vi "check_min_max_rules.vi"(10 "rules list":string[][](array[string])) -> (0 "empty/wrong?":bool=TRUE, 1 "message":string, 2 "min_length":string, 3 "max_length":string)   [LabVIEW 2024]
panel:
  # "max"
  # "min"
  # "lit when empty/wrong"
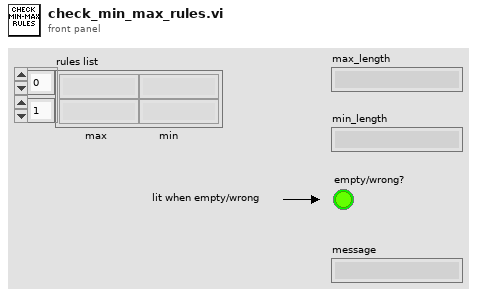
[diagram p1: front panel]
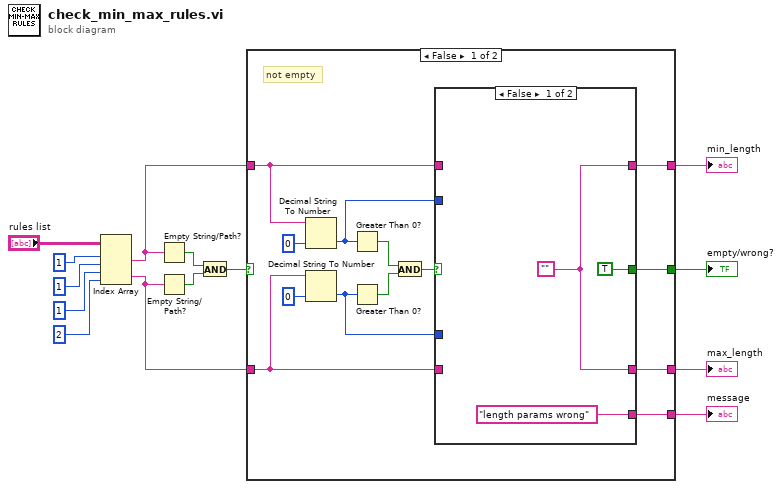
[diagram p0: block diagram]
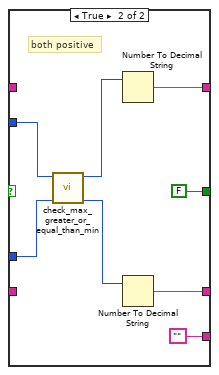
[diagram p2: hidden frame]
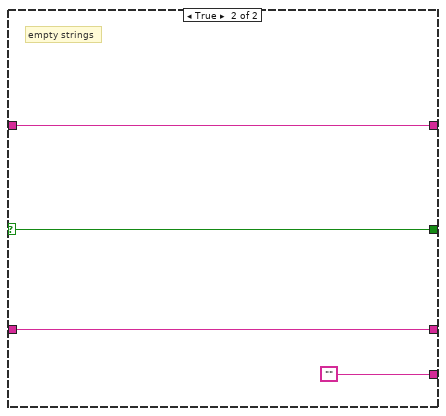
[diagram p3: hidden frame]
diagram:
  n1 = Index Array(array="rules list", index (row) #1=1 ("index"), index (col) #1=1 ("index"), index (row) #2=1 ("index"), index (col) #2=2 ("index")) -> (element #1=w9:string, element #2=w8:string)
  n2 = Empty String/Path?(string/path=w9) -> (empty?=w12:bool)
  n3 = Empty String/Path?(string/path=w8) -> (empty?=w11:bool)
  n4 = And(x=w12, y=w11) -> (x .and. y?=w10:bool)
  n5 = case shown="False" w10 {
    selector: w10 -> [_ w41]
    tunnel: w9 -> [w19 w40]
    tunnel: w8 -> [w18 w39]
    tunnel: [w20 ""] -> w7
    tunnel: [w17 w41] -> w6
    tunnel: [w15 w40] -> w4
    tunnel: [w16 w39] -> w5
    frame False {
      # "not empty"
      n6 = Decimal String To Number(string=w19, default (0L)=u8 0 ("default (0 I32)")) -> (number=w23:u8)  [unwired: 1 in, 1 out]
      n7 = Decimal String To Number(string=w18, default (0L)=u8 0 ("default (0 I32)")) -> (number=w22:u8)  [unwired: 1 in, 1 out]
      n8 = Greater Than 0?(x=w23) -> (x > 0?=w25:bool)
      n9 = Greater Than 0?(x=w22) -> (x > 0?=w24:bool)
      n10 = And(x=w25, y=w24) -> (x .and. y?=w21:bool)
      n11 = case shown="False" w21 {
        tunnel: w23 -> [_ w37]
        tunnel: w22 -> [_ w33]
        tunnel: ["length params wrong" ""] -> w20
        tunnel: w19 -> [_ _]
        tunnel: [w29 w31] -> w15
        tunnel: w18 -> [_ _]
        tunnel: [w29 w34] -> w16
        tunnel: [TRUE FALSE] -> w17
        frame False {
          w29 = ""
        }
        frame True {
          # "both positive"
          n12 = call "check_max_greater_or_equal_than_min.vi"("max_len_in"=w33, "min_len_in"=w37) -> ("max_len_out"=w32:i8, "min_len_out"=w35:i8)  [unwired: 8 in]
          n13 = Number To Decimal String(number=w35) -> (decimal integer string=w31:string)  [unwired: 1 in]
          n14 = Number To Decimal String(number=w32) -> (decimal integer string=w34:string)  [unwired: 1 in]
        }
      }
    }
    frame True {
      # "empty strings"
    }
  }
  "message" <- w7
  "empty/wrong?" <- w6
  "max_length" <- w5
  "min_length" <- w4
